vi "Arguments - Complex Data As Arguments.vi"() -> ()   [LabVIEW 2014]
uses:
  user.lib/_NEVSTOP/JKI State Machine ++/JKI State Machine++.lvlib
panel:
  out "HEX String (0-9,A-F) 2":string="1400800000000002000D400300074E756D65726963001240400001FFFFFFFF0000054172726179000100010000000500000241000081790000002C000001640000002D00000000"
  out "HEX String (0-9,A-F)":string="1400800000000005000C40210673746174757300000B40030004636F64650000104030FFFFFFFF06736F757263650000104030FFFFFFFF06737472696E67000022405000040000000100020003136572726F7220696E20286E6F206572726F7229000100040100038BF000000033436865636B20596F757220496E7465726E65742053706565642077697468206F7572205370656564205465737420546F6F6C2000000033436865636B20596F757220496E7465726E65742053706565642077697468206F7572205370656564205465737420546F6F6C2000000000"
  out "Array 2":i32[](array[numeric])=[577, 33145, 44, 356, 45]
  in  "Array":i32[](array[numeric])=[577, 33145, 44, 356, 45]
  out "value":T1={"status"=TRUE, "code"=232432, "source"="Check Your Internet Speed with our Speed Test Tool ", "string"="Check Your Internet Speed with our Speed Test Tool "}
  in  "error in (no error)":T1={"status"=TRUE, "code"=232432, "source"="Check Your Internet Speed with our Speed Test Tool ", "string"="Check Your Internet Speed with our Speed Test Tool "}
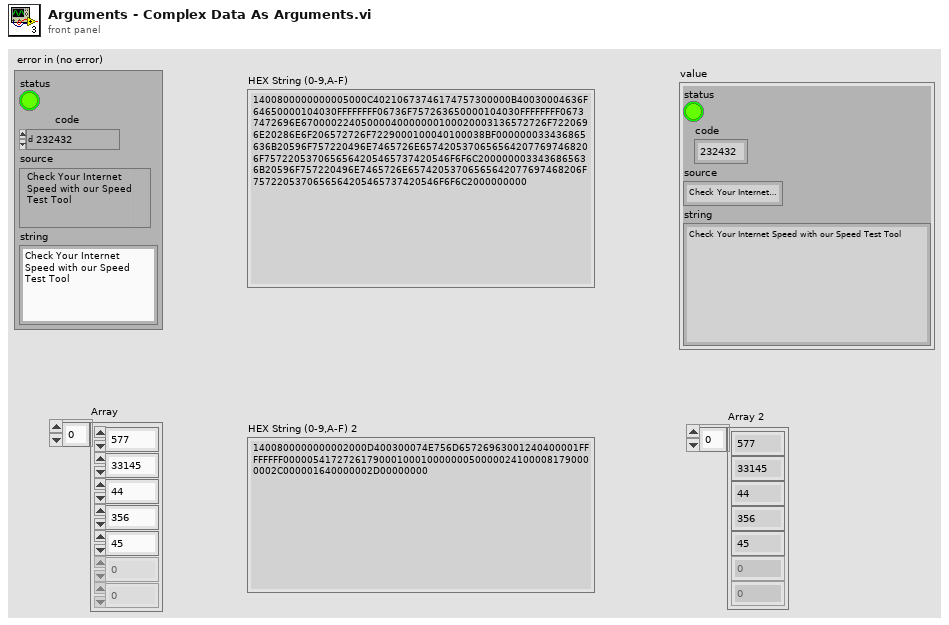
[diagram p1: front panel]
types:
  T1 = cluster{"status":bool, "code":i32, "source":string, "string":string}
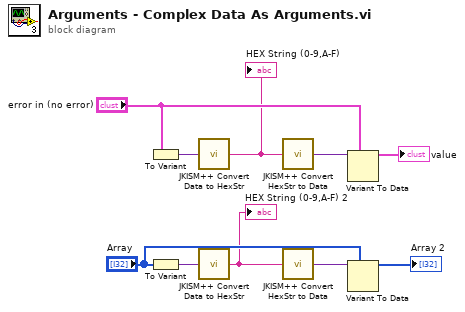
[diagram p0: block diagram]
diagram:
  n1 = To Variant(anything="error in (no error)") -> (Variant=w8:variant)
  n2 = To Variant(anything="Array") -> (Variant=w4:variant)
  n3 = call "JKISM++ Convert Data to HexStr.vi"("Variant"=w8) -> ("HEX String (0-9,A-F)"=w7:string)  [unwired: 8 in]
  "HEX String (0-9,A-F)" <- w7
  n4 = call "JKISM++ Convert Data to HexStr.vi"("Variant"=w4) -> ("HEX String (0-9,A-F)"=w1:string)  [unwired: 8 in]
  "HEX String (0-9,A-F) 2" <- w1
  n5 = call "JKISM++ Convert HexStr to Data.vi"("HEX String"=w7) -> ("Variant"=w6:variant)  [unwired: 8 in]
  n6 = call "JKISM++ Convert HexStr to Data.vi"("HEX String"=w1) -> ("Variant"=w5:variant)  [unwired: 8 in]
  n7 = Variant To Data(type="error in (no error)", Variant=w6) -> (data=→"value":T1)  [unwired: 1 in, 1 out]
  n8 = Variant To Data(type="Array", Variant=w5) -> (data=→"Array 2":i32[])  [unwired: 1 in, 1 out]
